vi "build_quaternion.vi"(8 "x":dbl[](array[numeric])=[0.0, 0.0, 0.0], 11 "w":dbl format="%.5f") -> (3 "Quaternion":dbl[](array[numeric]))   [LabVIEW 2013]
panel:
  # "Build a quaternion from components."
  # "w"
  # "x1"
  # "x2"
  # "x3"
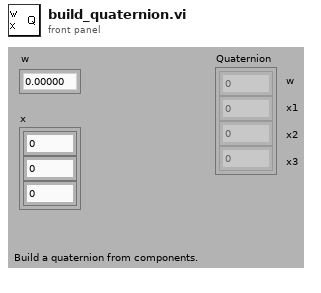
[diagram p1: front panel]
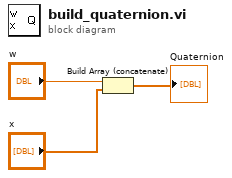
[diagram p0: block diagram]
diagram:
  n1 = Build Array (concatenate)("w", "x") -> (→"Quaternion":dbl[])
